vi "CTRE_CANTalonSRX_SetReference.vi"(6 "Reverse Closed-Loop Output":bool, 8 "error in (no error)":errorcluster, 9 "Reverse Feedback Sensor":bool, 10 "Feedback Reference":T1, 11 "CAN Talon SRX Ref":T2={"DeviceStatus"={"status"=FALSE, "code"=0, "source"=""}, "Type"=enum."PWM", "PWM"={"PWM Channel"=enum."PWM 1", "DeadBand"={"Name"="", "maxPositivePwm"=0, "minPositivePwm"=0, "centerPwm"=0, "maxNegativePwm"=0, "minNegativePwm"=0, "angularRange"=0}}, "CAN"={"Device Number"=0, "SetOutput VI Ref"=variant(enum8{"Percent VBus", "Current", "Speed", "Position", "Voltage"} enum."Percent VBus"), "GetOutput VI Ref"=variant(refnum<k1> refnum), "Enable VI Ref"=variant(dbl 12.0), "Disable VI Ref"=variant(enum8{"Percent VBus", "Speed", "Position", "Slave", "Unchanged / Invalid", "Voltage Compensation", "Current", "Motion Profile"} enum."Percent VBus"), "Data"=variant}, "Invert"=FALSE}) -> (0 "error out":errorcluster, 3 "CAN Talon SRX Ref":T2={"DeviceStatus"={"status"=FALSE, "code"=0, "source"=""}, "Type"=enum."PWM", "PWM"={"PWM Channel"=enum."PWM 1", "DeadBand"={"Name"="", "maxPositivePwm"=0, "minPositivePwm"=0, "centerPwm"=0, "maxNegativePwm"=0, "minNegativePwm"=0, "angularRange"=0}}, "CAN"={"Device Number"=0, "SetOutput VI Ref"=variant(enum8{"Percent VBus", "Current", "Speed", "Position", "Voltage"} enum."Percent VBus"), "GetOutput VI Ref"=variant(refnum<k1> refnum), "Enable VI Ref"=variant(dbl 12.0), "Disable VI Ref"=variant(enum8{"Percent VBus", "Speed", "Position", "Slave", "Unchanged / Invalid", "Voltage Compensation", "Current", "Motion Profile"} enum."Percent VBus"), "Data"=variant}, "Invert"=FALSE})   [LabVIEW 2016]
doc: "Select the sensor used as the position process variable for the PID controller.\n\n<B>Quad Encoder</B>: Selects a quadrature encoder.\n<B>Potentiometer</B>: Selects the analog input.\n<B>None</B>: No sensor selected.\n\n<B>Invert Closed-Loop Output</B> inverts the motor output when using closed-loop modes."
uses:
  <vilib>/Rock Robotics/WPI/MotorControl/WPI_MotorControlDeviceRef.ctl
  <vilib>/Rock Robotics/WPI/MotorControl/WPI_MotorControlType.ctl
  <vilib>/Rock Robotics/SystemInterfaces/DIO/FPGA_DIOPWMChannel.ctl
  <vilib>/Rock Robotics/WPI/PWM/WPI_PWMDeadband.ctl
  <vilib>/Rock Robotics/WPI/ThirdParty/CanMotor/CTRLib-LV-TalonSRX/WPI_CANTalonSRX_APIFeedbackSelect.ctl
  <vilib>/Rock Robotics/WPI/ThirdParty/CanMotor/CTRLib-LV-TalonSRX/CTRE_CANTalonSRX_FeedbackSelect.ctl
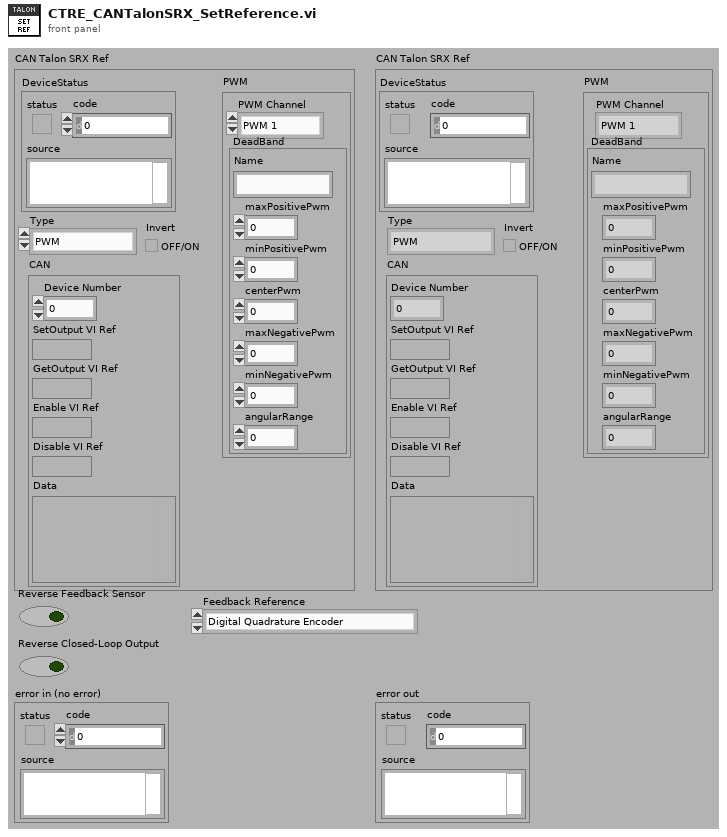
[diagram p1: front panel]
types:
  T1 = typedef "WPI_CANTalonSRX_APIFeedbackSelect.ctl" = enum16{"Digital Quadrature Encoder", "Analog Potentiometer", "Analog Encoder", "Count on Quad-A (Rising-Edge)", "Count on Quad-A (Falling-Edge)", "CTR Magnetic Enc (Absolute)", "CTR Magnetic Enc (Relative)", "Pulse Width"}
  T2 = typedef "WPI_MotorControlDeviceRef.ctl" = cluster{"DeviceStatus":errorcluster, "Type":T3, "PWM":cluster{"PWM Channel":T4, "DeadBand":T5}, "CAN":cluster{"Device Number":u8, "SetOutput VI Ref":variant, "GetOutput VI Ref":variant, "Enable VI Ref":variant, "Disable VI Ref":variant, "Data":variant}, "Invert":bool}
  T3 = typedef "WPI_MotorControlType.ctl" = enum16{"PWM", "CAN"}
  T4 = typedef "FPGA_DIOPWMChannel.ctl" = enum8{"PWM 0", "PWM 1", "PWM 2", "PWM 3", "PWM 4", "PWM 5", "PWM 6", "PWM 7", "PWM 8", "PWM 9", "PWM MXP 0", "PWM MXP 1", "PWM MXP 2", "PWM MXP 3", "PWM MXP 4", "PWM MXP 5", "PWM MXP 6", "PWM MXP 7", "PWM MXP 8", "PWM MXP 9", "Invalid"}
  T5 = typedef "WPI_PWMDeadband.ctl" = cluster{"Name":string, "maxPositivePwm":i32, "minPositivePwm":i32, "centerPwm":i32, "maxNegativePwm":i32, "minNegativePwm":i32, "angularRange":u16}
  T6 = typedef "CTRE_CANTalonSRX_FeedbackSelect.ctl" = u8
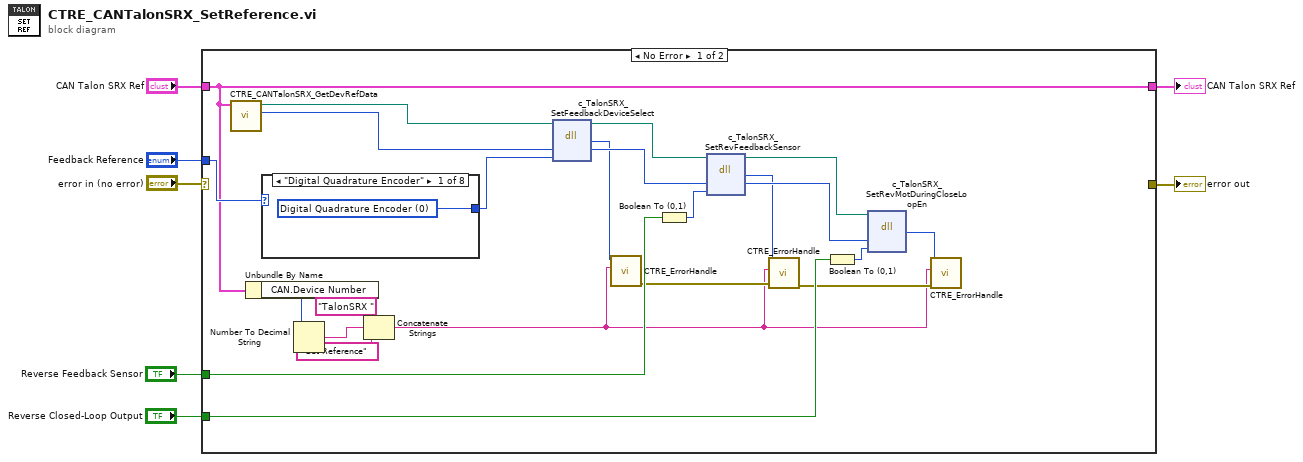
[diagram p0: block diagram]
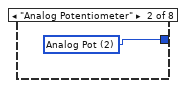
[diagram p2: hidden frame]
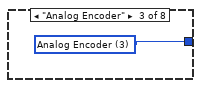
[diagram p3: hidden frame]
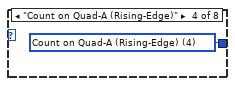
[diagram p4: hidden frame]
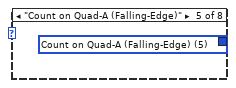
[diagram p5: hidden frame]
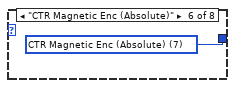
[diagram p6: hidden frame]
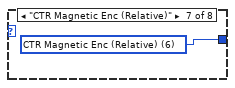
[diagram p7: hidden frame]
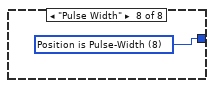
[diagram p8: hidden frame]
diagram:
  n1 = case shown="No Error" "error in (no error)" {
    selector: "error in (no error)" -> [_ w40]
    tunnel: [_ w40] -> w7
    tunnel: [w9 w39] -> w5
    tunnel: "CAN Talon SRX Ref" -> [w9 w39]
    tunnel: "Feedback Reference" -> [w30 _]
    tunnel: "Reverse Feedback Sensor" -> [w23 _]
    tunnel: "Reverse Closed-Loop Output" -> [w20 _]
    frame No Error {
      n2 = call <vilib>:"CTRE_CANTalonSRX_GetDevRefData.vi"("MotorControlDevRef"=w9) -> ("handle"=w27:u64, "Library"=w28:path)  [unwired: 6 in, 3 out]
      n3 = Unbundle By Name(w9) -> ("CAN.Device Number"=w10:u8)
      n4 = case shown="\"Digital Quadrature Encoder\"" w30 {
        tunnel: [w31 w32 w33 w34 w35 w36 w37 w38] -> w29
        frame "Digital Quadrature Encoder" {
          w31 = T6 0 items=["Digital Quadrature Encoder"=0, "Analog Pot"=2, "Analog Encoder"=3, "Count on Quad-A (Rising-Edge)"=4, "Count on Quad-A (Falling-Edge)"=5, "Position is Pulse-Width"=8] ("Talon SRX Feedback Select")
        }
        frame "Analog Potentiometer" {
          w32 = T6 2 items=["Digital Quadrature Encoder"=0, "Analog Pot"=2, "Analog Encoder"=3, "Count on Quad-A (Rising-Edge)"=4, "Count on Quad-A (Falling-Edge)"=5, "Position is Pulse-Width"=8] ("Talon SRX Feedback Select")
        }
        frame "Analog Encoder" {
          w33 = T6 3 items=["Digital Quadrature Encoder"=0, "Analog Pot"=2, "Analog Encoder"=3, "Count on Quad-A (Rising-Edge)"=4, "Count on Quad-A (Falling-Edge)"=5, "Position is Pulse-Width"=8] ("Talon SRX Feedback Select")
        }
        frame "Count on Quad-A (Rising-Edge)" {
          w34 = T6 4 items=["Digital Quadrature Encoder"=0, "Analog Pot"=2, "Analog Encoder"=3, "Count on Quad-A (Rising-Edge)"=4, "Count on Quad-A (Falling-Edge)"=5, "Position is Pulse-Width"=8] ("Talon SRX Feedback Select")
        }
        frame "Count on Quad-A (Falling-Edge)" {
          w35 = T6 5 items=["Digital Quadrature Encoder"=0, "Analog Pot"=2, "Analog Encoder"=3, "Count on Quad-A (Rising-Edge)"=4, "Count on Quad-A (Falling-Edge)"=5, "Position is Pulse-Width"=8] ("Talon SRX Feedback Select")
        }
        frame "CTR Magnetic Enc (Absolute)" {
          w36 = T6 7 items=["Digital Quadrature Encoder"=0, "Analog Pot"=2, "Analog Encoder"=3, "Count on Quad-A (Rising-Edge)"=4, "Count on Quad-A (Falling-Edge)"=5, "Position is Pulse-Width"=8, "CTR Magnetic Enc (Relative)"=6, "CTR Magnetic Enc (Absolute)"=7] ("Talon SRX Feedback Select")
        }
        frame "CTR Magnetic Enc (Relative)" {
          w37 = T6 6 items=["Digital Quadrature Encoder"=0, "Analog Pot"=2, "Analog Encoder"=3, "Count on Quad-A (Rising-Edge)"=4, "Count on Quad-A (Falling-Edge)"=5, "Position is Pulse-Width"=8, "CTR Magnetic Enc (Relative)"=6, "CTR Magnetic Enc (Absolute)"=7] ("Talon SRX Feedback Select")
        }
        frame "Pulse Width" {
          w38 = T6 8 items=["Digital Quadrature Encoder"=0, "Analog Pot"=2, "Analog Encoder"=3, "Count on Quad-A (Rising-Edge)"=4, "Count on Quad-A (Falling-Edge)"=5, "Position is Pulse-Width"=8] ("Talon SRX Feedback Select")
        }
      }
      n5 = Number To Decimal String(number=w10) -> (decimal integer string=w12:string)  [unwired: 1 in]
      n6 = Concatenate Strings("TalonSRX " ("string"), w12, " Set Reference" ("string")) -> (w8:string)
      n7 = dll-call lib="?" fn="c_TalonSRX_SetFeedbackDeviceSelect"(path in=w28, "handle"=w27, "param"=w29) -> (path out=w26:path, "return type"=w16:i32, "handle"=w25:u64)  [unwired: 3 in, 1 out]
      n8 = call <vilib>:"CTRE_ErrorHandle.vi"("origin"=w8, "code"=w16) -> ("error out"=w18:errorcluster)  [unwired: 9 in]
      n9 = Boolean To (0,1)(Boolean=w23) -> (0, 1=w24:i16)
      n10 = dll-call lib="?" fn="c_TalonSRX_SetRevFeedbackSensor"(path in=w26, "handle"=w25, "param"=w24) -> (path out=w22:path, "return type"=w15:i32, "handle"=w21:u64)  [unwired: 3 in, 1 out]
      n11 = call <vilib>:"CTRE_ErrorHandle.vi"("error in"=w18, "origin"=w8, "code"=w15) -> ("error out"=w17:errorcluster)  [unwired: 8 in]
      n12 = Boolean To (0,1)(Boolean=w20) -> (0, 1=w19:i16)
      n13 = dll-call lib="?" fn="c_TalonSRX_SetRevMotDuringCloseLoopEn"(path in=w22, "handle"=w21, "param"=w19) -> ("return type"=w14:i32)  [unwired: 4 in, 2 out]
      n14 = call <vilib>:"CTRE_ErrorHandle.vi"("error in"=w17, "origin"=w8, "code"=w14) -> ()  [unwired: 8 in, 1 out]
    }
    frame Error {
    }
  }
  "CAN Talon SRX Ref" <- w5
  "error out" <- w7
